vi "string contains substring.vi"(1 "Search String":string, 2 "Input String":string) -> (0 "Found?":bool)   [LabVIEW 2021]
uses:
  <vilib>/GPower/String/GPString.lvlib
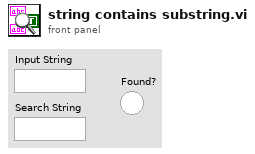
[diagram p1: front panel]
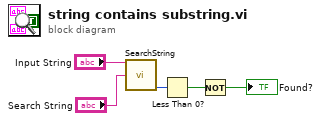
[diagram p0: block diagram]
diagram:
  n1 = call <vilib>:"SearchString.vi"("String"="Input String", "Search string"="Search String") -> ("Offset past match"=w3:i32)  [unwired: 11 in, 2 out]
  n2 = Less Than 0?(x=w3) -> (x < 0?=w2:bool)
  n3 = Not(x=w2) -> (.not. x?=→"Found?":bool)
